vi "sub_re-sampling.vi"(10 "pw":T1, 11 "px":T1) -> (2 "pw":T1, 3 "px out":T1)   [LabVIEW 2019]
uses:
  <vilib>/Analysis/Matrix/Datatypes/RealMatrix.ctl
  Ctrl/cmd_common.ctl
  <vilib>/Analysis/Matrix/Numeric/Add/Add (Elementwise) - RM,R.vi
  <vilib>/Analysis/Matrix/NI_Matrix.lvlib
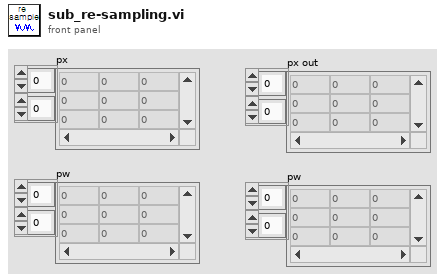
[diagram p1: front panel]
types:
  T1 = typedef "NI_Matrix.lvlib/RealMatrix.ctl" = dbl[][]
  T2 = typedef "cmd_common.ctl" = enum16{"read", "write"}
  T3 = cluster{"DT":dbl, "SIM_TIME":dbl, "MAX_RANGE":dbl, "NP":u32, "NTh":u32, "Q":T1, "R":T1, "Q_sim":T1, "R_sim":T1, "rf_id":cluster{"x":dbl, "y":dbl}[]}
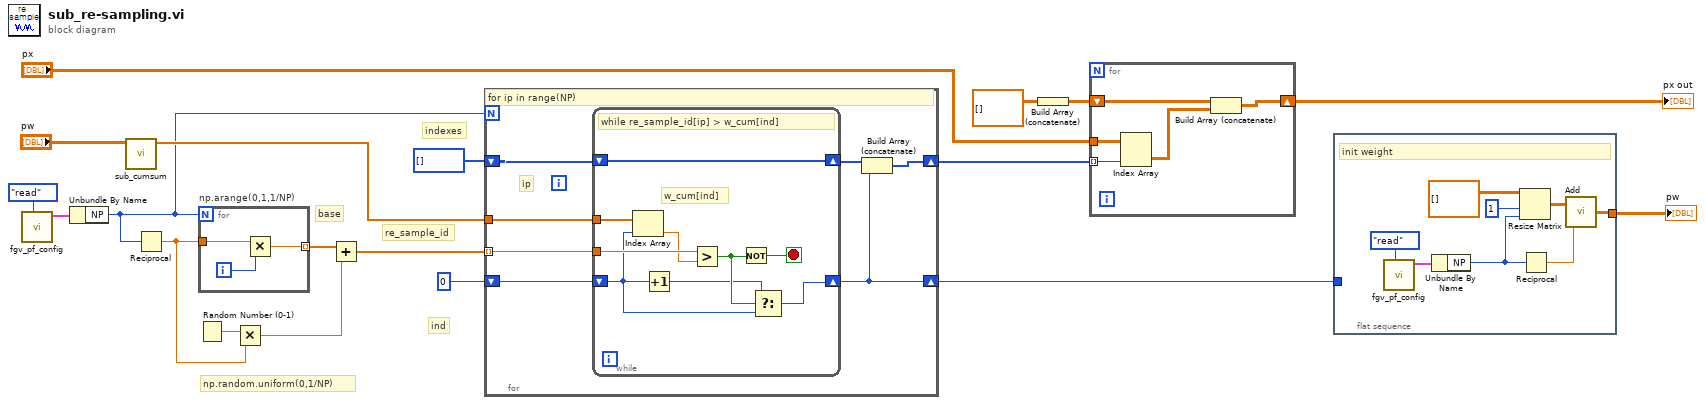
[diagram p0: block diagram]
diagram:
  # "indexes"
  # "ind"
  # "np.random.uniform(0,1/NP)"
  # "base"
  # "re_sample_id"
  n1 = call "fgv_pf_config.vi"("cmd"=cmd_common."read") -> ("pf-val out"=w4:T3)  [unwired: 10 in]
  n2 = Unbundle By Name(w4) -> ("NP"=w9:u32)
  n3 = call "sub_cumsum.vi"("in mat"="pw") -> ("cumsum"=w10:dbl[])  [unwired: 10 in]
  n4 = Reciprocal(x=w9) -> (1/x=w6:dbl)
  n5 = Random Number (0-1)() -> (number: 0 to 1=w5:dbl)
  n6 = for "np.arange(0,1,1/NP)" {
    N: w9 -> [_]
    tunnel: w6 -> [w21]
    tunnel: [w20] -> w8 mode=indexing
    i -> [w22]
    n7 = Multiply(x=w21, y=w22) -> (x*y=w20:dbl)
  }
  n8 = Multiply(x=w5, y=w6) -> (x*y=w7:dbl)
  n9 = Add(x=w8, y=w7) -> (x+y=w11:dbl[])
  n10 = for {
    N: w9 -> [_]
    tunnel: w11 -> [w29] mode=indexing
    tunnel: w10 -> [w28]
    shift-right: [w23] -> w1
    shift-left: 0 -> [w27]
    shift-right: [w24] -> w14
    shift-left: u64[] [] ("cumsum") -> [w26]
    # "ip"
    # "for ip in range(NP)"
    n11 = while {
      tunnel: w29 -> [w36]
      tunnel: w28 -> [w37]
      shift-right: [w38] -> w25
      shift-left: w26 -> [w38]
      shift-right: [w30] -> w23
      shift-left: w27 -> [w32]
      stop <- w34 stop-if-true
      # "w_cum[ind]"
      # "while re_sample_id[ip] > w_cum[ind]"
      n12 = Index Array(array=w37, index=w32) -> (element=w35:dbl)
      n13 = Increment(x=w32) -> (x+1=w31:i32)
      n14 = Greater?(x=w36, y=w35) -> (0:w33:bool)
      n15 = Not(x=w33) -> (.not. x?=w34:bool)
      n16 = Select(t=w31, s=w33, f=w32) -> (s? t:f=w30:i32)
    }
    n17 = Build Array (concatenate)(w25, w23) -> (w24:u64[])
  }
  n18 = Build Array (concatenate)(dbl[][] []) -> (w16:T1)
  n19 = for {
    tunnel: w14 -> [w40] mode=indexing
    tunnel: "px" -> [w41]
    shift-right: [w42] -> w18
    shift-left: w16 -> [w43]
    n20 = Index Array(array=w41, index (col)=w40) -> (element=w39:T1)  [unwired: 1 in]
    n21 = Build Array (concatenate)(w43, w39) -> (w42:T1)
  }
  "px out" <- w18
  n22 = flat-sequence {
    tunnel: [w51] -> w19
    tunnel: w1 -> [_]
    frame #0 {
      # "init weight"
      n23 = call "fgv_pf_config.vi"("cmd"=cmd_common."read") -> ("pf-val out"=w44:T3)  [unwired: 10 in]
      n24 = Unbundle By Name(w44) -> ("NP"=w50:u32)
      n25 = Resize Matrix(1:w50, 2:1 ("행의 개수"), 4:T1 [] ("행렬")) -> (0:w45:T1)
      n26 = Reciprocal(x=w50) -> (1/x=w46:dbl)
      n27 = call-poly <vilib>:"Add.vi"("Real Scalar c"=w46, "Real Matrix A"=w45) -> ("A + c"=w51:T1)
    }
  }
  "pw" <- w19
